vi "GetSubPanelRef.vi"(6 "timeout in ms (-1)":i32, 8 "error in (no error)":errorcluster, 11 "EmbeddedSMO in":refnum<class "EmbeddedSMO.lvclass">) -> (0 "error out":errorcluster, 2 "SubPanelReference":refnum<vi>, 3 "EmbeddedSMO out":refnum<class "EmbeddedSMO.lvclass">)   [LabVIEW 2016, in "EmbeddedSMO.lvclass"]
uses:
  EmbeddedSMO.lvclass
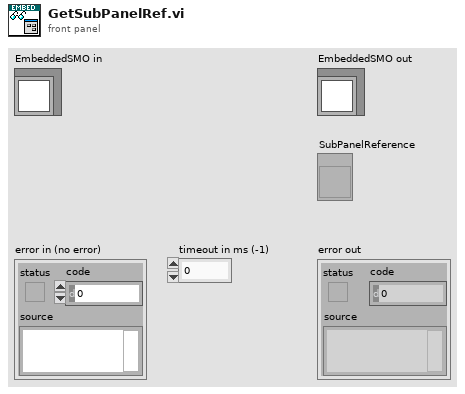
[diagram p1: front panel]
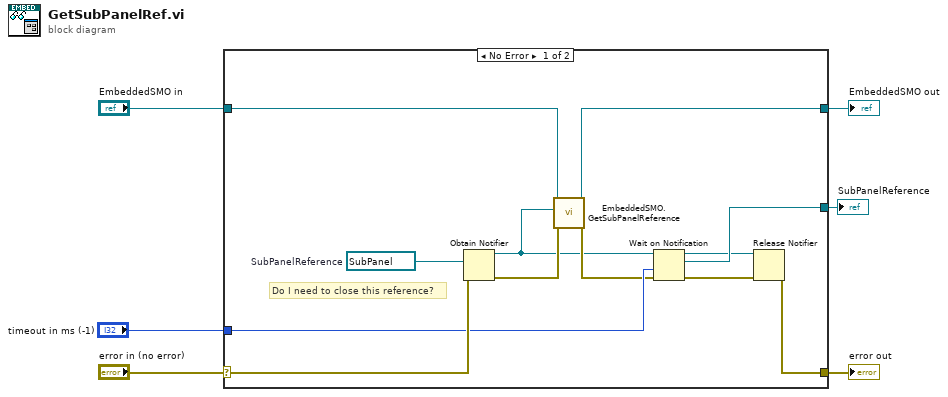
[diagram p0: block diagram]
diagram:
  n1 = case shown="No Error" "error in (no error)" {
    selector: "error in (no error)" -> [w13 w20]
    tunnel: [w14 w20] -> w5
    tunnel: [w7 w19] -> w3
    tunnel: "EmbeddedSMO in" -> [w8 w19]
    tunnel: [w17 _] -> w2
    tunnel: "timeout in ms (-1)" -> [w12 _]
    frame No Error {
      w18 = refnum<vi> refnum  # SubPanelReference
      # "Do I need to close this reference?"
      n2 = Obtain Notifier(notification data type=w18, error in (no error)=w13) -> (notifier out=w9:refnum<notifier>, error out=w10:errorcluster)  [unwired: 2 in, 1 out]
      n3 = call "EmbeddedSMO.GetSubPanelReference.vi"("error in (no error)"=w10, "GetSubPanelReference"=w9, "EmbeddedSMO"=w8) -> ("error out"=w11:errorcluster, "EmbeddedSMO out"=w7:refnum<class "EmbeddedSMO.lvclass">)  [unwired: 7 in]
      n4 = Wait on Notification(notifier=w9, timeout in ms (-1)=w12, error in (no error)=w11) -> (notifier out=w16:refnum<notifier>, notification=w17:refnum<vi>, error out=w15:errorcluster)  [unwired: 1 in, 1 out]
      n5 = Release Notifier(notifier=w16, error in (no error)=w15) -> (error out=w14:errorcluster)  [unwired: 1 in, 2 out]
    }
    frame Error {
    }
  }
  "error out" <- w5
  "EmbeddedSMO out" <- w3
  "SubPanelReference" <- w2
